vi "MakeSurviveCycleCode.vi"(11 "TestCycleParameters":T1={"TAmb"=20.0, "HeaterTestTemp"=-80.0, "HeaterTestDwell(min)"=30, "HeaterTestDuration"=15, "MinOpTemp"=-50.0, "MinOpDwell(min)"=30, "TestHeatingRate (deg/min)"=0.4, "SurviveCycleParameters"={"MinSurviveTemp"=-131.5, "MinSurvive Dwell(min)"=10, "MaxSurviveTemp"=50.0, "MaxSurviveDwell(min)"=30, "ControlInput"=2, "ColdStandOff"=4.0, "HotStandoff"=5.0, "SteadyPWM"=20, "MaxCoolingRate (deg/min)"=3.75, "MaxHeatingRate (deg/min)"=2.5}, "CycleType"=0, "MaxOpTemp"=-50.0, "MaxOpDwell(min)"=30} {"CycleType" items=["Survival", "Operational"]; "SurviveCycleParameters"."SteadyPWM" min=0 max=100 step=1; "SurviveCycleParameters"."ControlInput" items=["3A", "3B", "3C", "3D", "4A", "4B", "4C", "4D"]}) -> (1 "Profile":cluster{dbl[], dbl[]}(graph)={[0.0, 25.0, 85.0, 97.5, 127.5, 142.5, 150.0, 180.0, 430.0, 460.0], [20.0, -130.0, -130.0, -80.0, -80.0, -80.0, -50.0, -50.0, 50.0, 50.0]}, 3 "resulting string":string="define onecycle (pwm=100 run pwmloop 5A.PID.Setpoint=-131.500000  while(#3C >-129.5){pause 0.2 s}pwm=10 pause 10 min kill pwmloop pwm=0 relays=0 5A.PID.SetPoint=51.0 while(#3C<50.0){pause 0.2 s} pause 10 min)")   [LabVIEW 2024]
uses:
  controls/TestCycleParams.ctl
  controls/SurviveCycleParams.ctl
  controls/ControlInput.ctl
panel:
  in  "Tab Control":enum32{"Profile", "Code"}(tab)
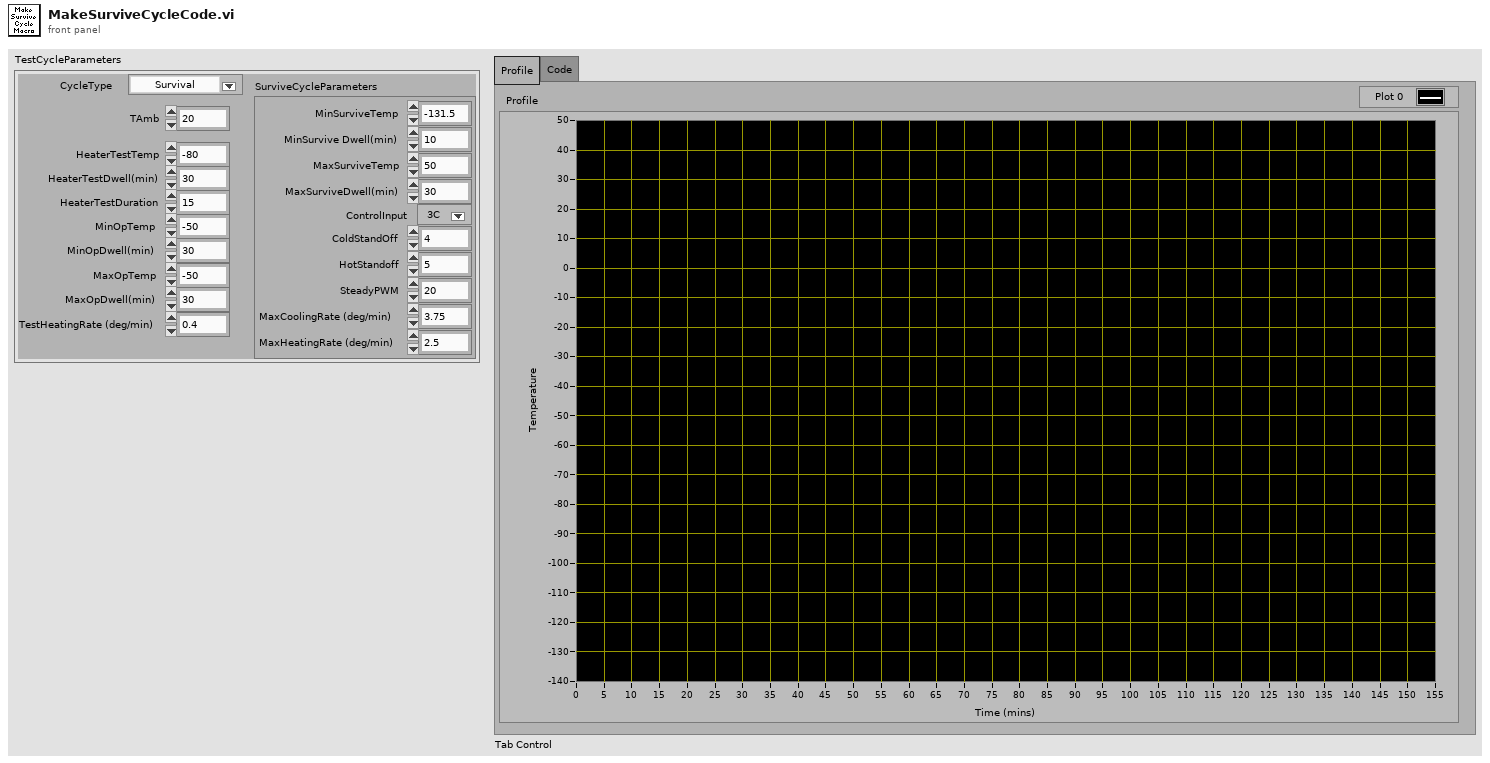
[diagram p1: front panel]
types:
  T1 = typedef "TestCycleParams.ctl" = cluster{"TAmb":dbl, "HeaterTestTemp":dbl, "HeaterTestDwell(min)":i32, "HeaterTestDuration":i32, "MinOpTemp":dbl, "MinOpDwell(min)":i32, "TestHeatingRate (deg/min)":dbl, "SurviveCycleParameters":T2, "CycleType":u16, "MaxOpTemp":dbl, "MaxOpDwell(min)":i32}
  T2 = typedef "SurviveCycleParams.ctl" = cluster{"MinSurviveTemp":dbl, "MinSurvive Dwell(min)":i32, "MaxSurviveTemp":dbl, "MaxSurviveDwell(min)":i32, "ControlInput":T3, "ColdStandOff":dbl, "HotStandoff":dbl, "SteadyPWM":i32, "MaxCoolingRate (deg/min)":dbl, "MaxHeatingRate (deg/min)":dbl}
  T3 = typedef "ControlInput.ctl" = u16
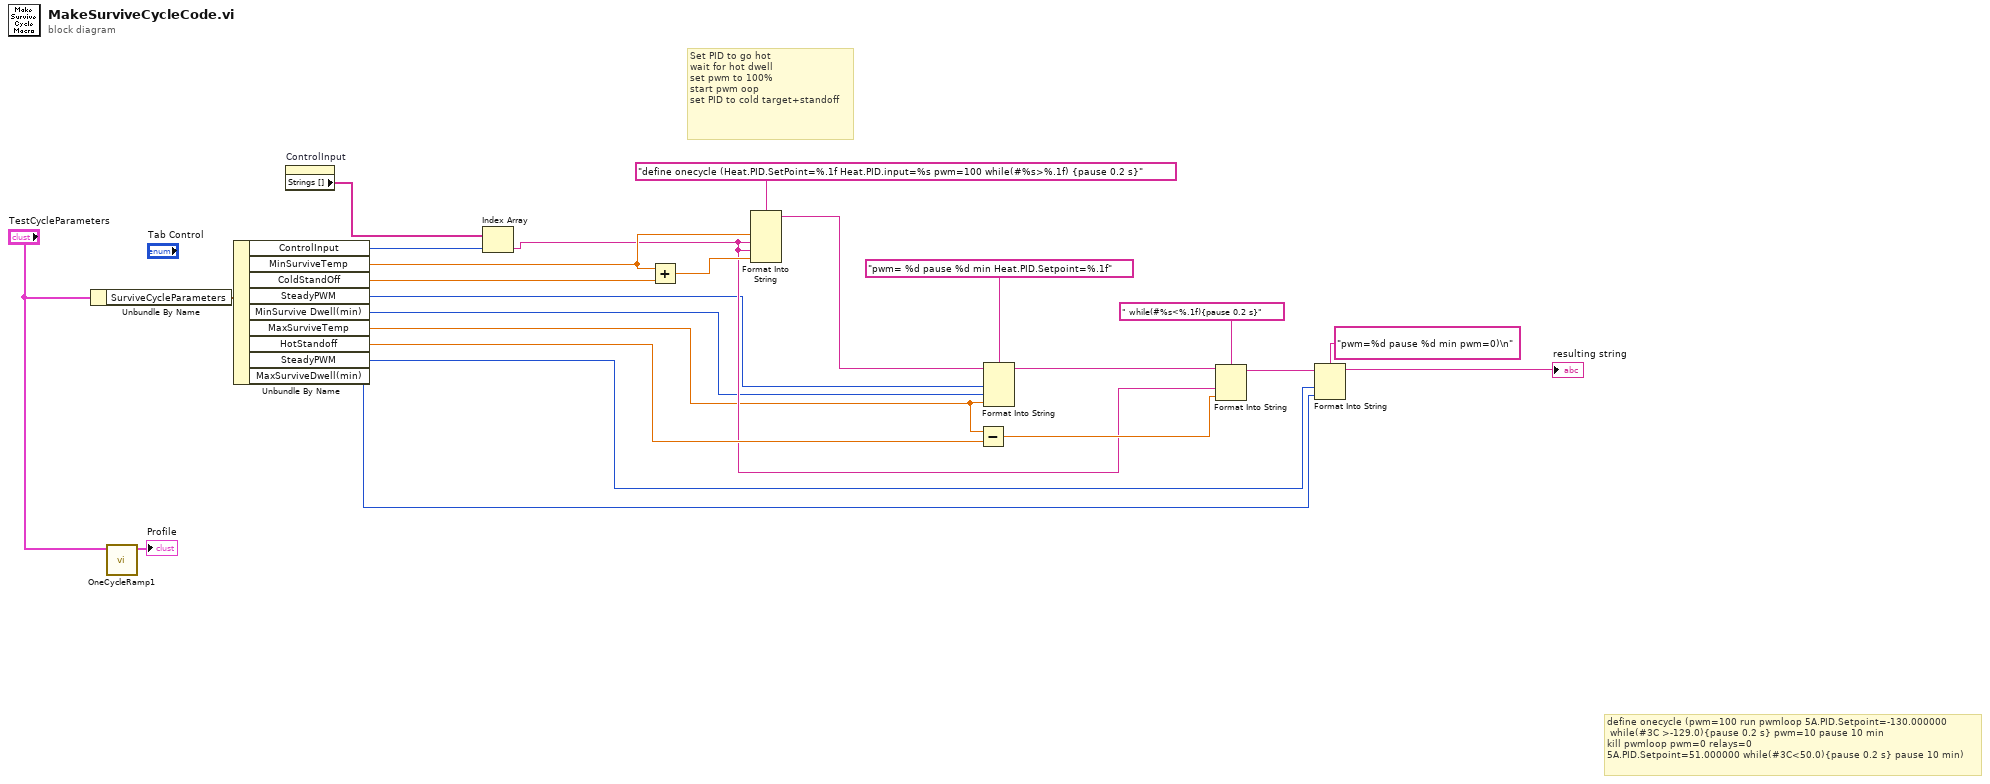
[diagram p0: block diagram]
diagram:
  # "Set PID to go hot\nwait for hot dwell\nset pwm to 100%\nstart pwm oop\nset PID to cold target+standoff"
  # "define onecycle (pwm=100 run pwmloop 5A.PID.Setpoint=-130.000000\n while(#3C >-129.0){pause 0.2 s} pwm=10 pause 10 min \nkill pwmloop pwm=0 relays=0 \n5A.PID.Setpoint=51.000000 while(#3C<50.0){pause 0.2 s} pause 10 min)"
  n1 = Unbundle By Name("TestCycleParameters") -> ("SurviveCycleParameters"=w8:T2)
  n2 = call "OneCycleRamp1.vi"("TestCycleParameters"="TestCycleParameters") -> ("Profile"=→"Profile":cluster{dbl[], dbl[]})  [unwired: 10 in]
  n3 = Unbundle By Name(w8) -> ("ControlInput"=w9:T3, "MinSurviveTemp"=w14:dbl, "ColdStandOff"=w13:dbl, "SteadyPWM"=w3:i32, "MinSurvive Dwell(min)"=w1:i32, "MaxSurviveTemp"=w2:dbl, "HotStandoff"=w12:dbl, "SteadyPWM"=w11:i32, "MaxSurviveDwell(min)"=w10:i32)
  n4 = property on="ControlInput" class="Ring (strict)"() -> ("Strings []"=w6:string[])  [unwired: 2 in, 2 out]
  n5 = Index Array(array=w6, index=w9) -> (element=w7:string)
  n6 = Add(x=w14, y=w13) -> (x+y=w23:dbl)
  n7 = Format Into String(format string="define onecycle (Heat.PID.SetPoint=%.1f Heat.PID.input=%s pwm=100 while(#%s>%.1f) {pause 0.2 s}", w14, w7, w7, w23) -> (resulting string=w18:string)  [unwired: 2 in, 1 out]
  n8 = Subtract(x=w2, y=w12) -> (x-y=w17:dbl)
  n9 = Format Into String(format string="pwm= %d pause %d min Heat.PID.Setpoint=%.1f", initial string=w18, w3, w1, w2) -> (resulting string=w19:string)  [unwired: 1 in, 1 out]
  n10 = Format Into String(format string=" while(#%s<%.1f){pause 0.2 s}", initial string=w19, w7, w17) -> (resulting string=w16:string)  [unwired: 1 in, 1 out]
  n11 = Format Into String(format string="pwm=%d pause %d min pwm=0)\n", initial string=w16, w11, w10) -> (resulting string=→"resulting string":string)  [unwired: 1 in, 1 out]
